vi "dP_data_labels.vi"() -> (0 "dP Data Labels":string[](array[string])=["Timestamp", "Vap Mass Flow", "Liq Mass Flow", "DP", "Liq Tank P", "LiqTank T", "Sep P", "SepT", "Liq In P", "Liq In T", "Vap Tank P", "Vap Tank T", "Dev Section P", "Dev Section T", "Up TS P", "Up TS T", "Low TS P", "Low TS T", "Cond Top T", "Evap Top T", "Cond Bot T", "Evap Bot T", "Win 3-4 P", "Top Heat T", "Bot Heat T", ""])   [LabVIEW 2017]
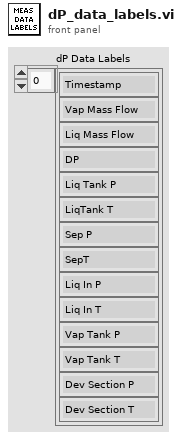
[diagram p1: front panel]
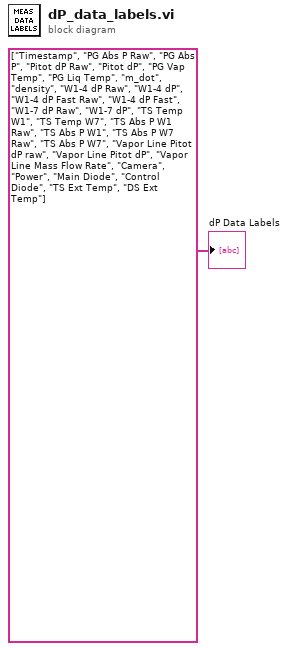
[diagram p0: block diagram]
diagram:
  "dP Data Labels" <- string[] ["Timestamp", "PG Abs P Raw", "PG Abs P", "Pitot dP Raw", "Pitot dP", "PG Vap Temp", "PG Liq Temp", "m_dot", "density", "W1-4 dP Raw", "W1-4 dP", "W1-4 dP Fast Raw", "W1-4 dP Fast", "W1-7 dP Raw", "W1-7 dP", "TS Temp W1", "TS Temp W7", "TS Abs P W1 Raw", "TS Abs P W1", "TS Abs P W7 Raw", "TS Abs P W7", "Vapor Line Pitot dP raw", "Vapor Line Pitot dP", "Vapor Line Mass Flow Rate", "Camera", "Power", "Main Diode", "Control Diode", "TS Ext Temp", "DS Ext Temp"]
